vi "Patch data preview prototype.vi"(11 "Dataset path":path=path "C:/Users/Teo/Desktop/UCL Datasets/160915_13_48_57 FunctAcq-6 patches") -> ()   [LabVIEW 2017]
uses:
  Patch data preview/Typedefs/Patch viewer states.ctl
  Typedefs/Read Write Enum.ctl
panel:
  in  "Channel to load":enum16{"Red", "Green"}(ring)
  out "Slider at trial #":i32=11 format="Cycle: %.0f"
  in  "Scrollbar":i32(c297)=11
  out "Image":T1(plugin-control)
  in  "Number of rows to generate":i32=3
  # "C:\\Users\\Teo\\Desktop\\UCL Datasets\\160408_12_51_00-backwards jumps-Patches"
  # "This is the prototype patch data preview window. Its functionality will be integrated in the \"Window-Functional data editor.vi\"\nUpgrade to handle datasets with multiple trials."
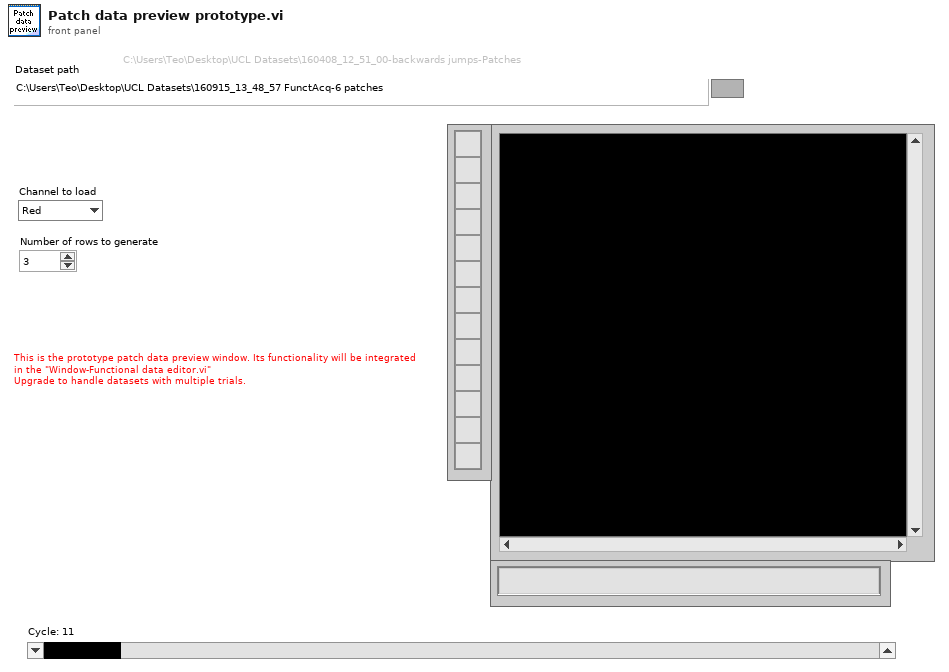
[diagram p1: front panel]
types:
  T1 = typedef "IMAQ Image.ctl" = refnum<image>
  T2 = typedef "Patch viewer states.ctl" = enum16{"Initialise", "Refresh", "Idle", "Error"}
  T3 = typedef "Read Write Enum.ctl" = enum16{"Read", "Write"}
  T4 = typedef "Patch viewer internal cluster.ctl" = cluster{"Image ref":T1, "Coordinates of montage positions":cluster{"X\n\nY":i32[]}[], "TDMS refs":refnum<k34>[], "Frames info":cluster{"Frame numbers used":i32[], "Frame position index":i32[]}, "Number of trials":i32, "Cycles in single trial":i32, "Total number of cycles":i32, "Number of patches":i32, "Pixels in a cycle":i32, "Patches info array":cluster{"Pixels in a patch":i32, "X size of patch":i32, "Y size of patch":i32}[], "error":errorcluster}
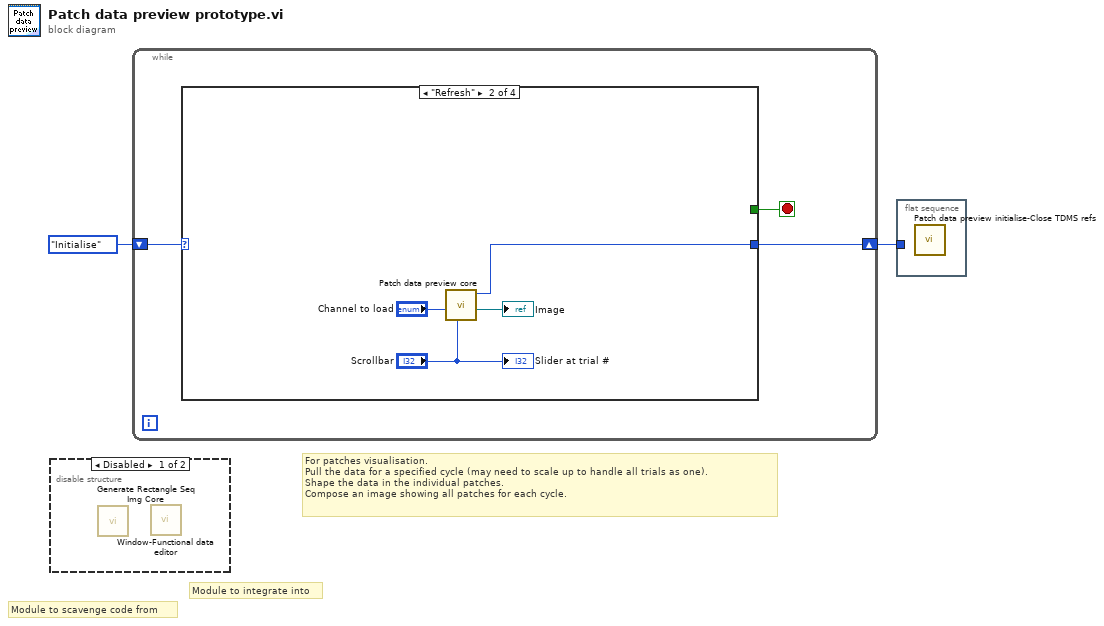
[diagram p0: block diagram]
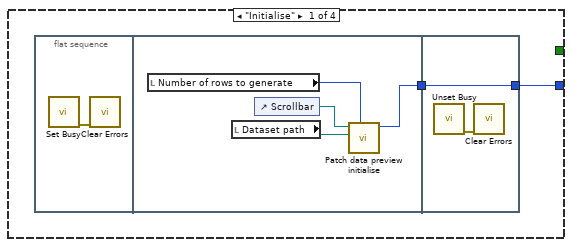
[diagram p3: hidden frame]
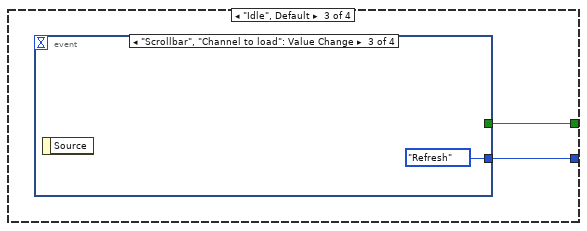
[diagram p4: hidden frame]
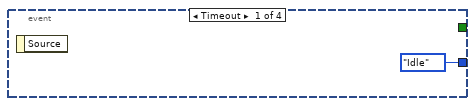
[diagram p5: hidden frame]
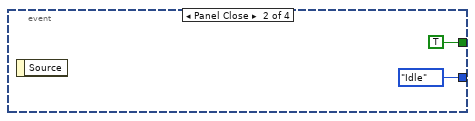
[diagram p6: hidden frame]
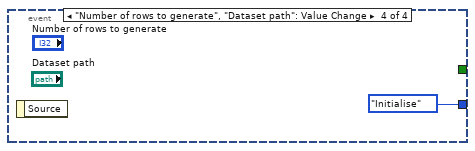
[diagram p7: hidden frame]
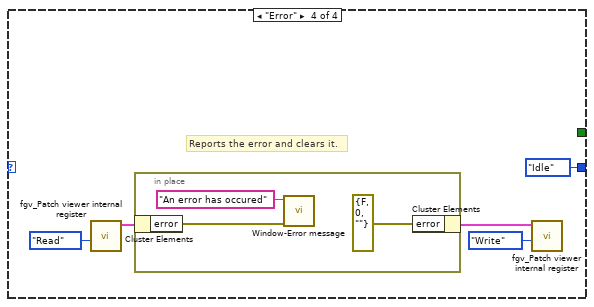
[diagram p8: hidden frame]
diagram:
  # "Module to integrate into"
  # "Module to scavenge code from"
  # "For patches visualisation.\nPull the data for a specified cycle (may need to scale up to handle all trials as one).\nShape the data in the individual patches.\nCompose an image showing all patches for each cycle."
  n1 = disable-structure shown="Disabled" {
    frame Disabled {
      n2 = call "Generate Rectangle Seq Img Core.vi"() -> ()  [unwired: 10 in, 2 out]
      n3 = call "Window-Functional data editor.vi"() -> ()  [unwired: 12 in]
    }
    frame Enabled {
    }
  }
  n4 = while {
    shift-right: [w3] -> w1
    shift-left: Patch_viewer_states."Initialise" ("States") -> [w5]
    stop <- w4 stop-if-true
    n5 = case shown="\"Refresh\"" w5 {
      tunnel: [_ _ w20 _] -> w4
      tunnel: [w7 w16 w19 Patch_viewer_states."Idle" ("States")] -> w3
      frame "Initialise" {
        n6 = flat-sequence {
          tunnel: [w10] -> w6
          tunnel: [w14] -> w7
          tunnel: w6 -> [w14]
          frame #0 {
            n7 = call <vilib>:"Set Busy.vi"() -> ("error out"=w8:errorcluster)  [unwired: 10 in, 1 out]
            n8 = call <vilib>:"Clear Errors.vi"("error in (no error)"=w8) -> ()  [unwired: 5 in, 2 out]
          }
          frame #1 {
            n9 = local read "Number of rows to generate"() -> (w9:i32)
            n10 = local read "Dataset path"() -> (w11:path)
            n11 = control-ref of="Scrollbar"() -> (w12:refnum<vi>)
            n12 = call "Patch data preview initialise.vi"("Number of rows to generate"=w9, "Dataset path"=w11, "Scrollbar ref"=w12) -> ("Next state"=w10:T2)  [unwired: 8 in]
          }
          frame #2 {
            n13 = call <vilib>:"Unset Busy.vi"() -> ("error out"=w13:errorcluster)  [unwired: 11 in]
            n14 = call <vilib>:"Clear Errors.vi"("error in (no error)"=w13) -> ()  [unwired: 5 in, 2 out]
          }
        }
      }
      frame "Refresh" {
        n15 = call "Patch data preview core.vi"("Global cycle number among all trials"="Scrollbar", "Channel to load"="Channel to load") -> ("Image ref (montage)"=→"Image":T1, "Next state"=w16:T2)  [unwired: 8 in]
        "Slider at trial #" <- "Scrollbar"
      }
      frame "Idle", Default {
        n16 = event shown="[2] \"Scrollbar\", \"Channel to load\": Value Change" {
          selector: _ -> [_ _ _ _]
          dyn-events: _ -> [_ _ _ _]
          timeout: _ -> [_ _ _ _]
          tunnel: [_ TRUE _ _] -> w20
          tunnel: [Patch_viewer_states."Idle" ("States") Patch_viewer_states."Idle" ("States") Patch_viewer_states."Refresh" ("States") Patch_viewer_states."Initialise" ("States")] -> w19
          event Timeout {
            n17 = event-data() -> ()  [unwired: 1 in, 1 out]
          }
          event Panel Close {
            n18 = event-data() -> ()  [unwired: 1 in, 1 out]
          }
          event "Scrollbar", "Channel to load": Value Change {
            n19 = event-data() -> ()  [unwired: 1 in, 1 out]
          }
          event "Number of rows to generate", "Dataset path": Value Change {
            n20 = event-data() -> ()  [unwired: 1 in, 1 out]
          }
        }
      }
      frame "Error" {
        # "Reports the error and clears it."
        n21 = call "fgv_Patch viewer internal register.vi"("Function"=Read_Write_Enum."Read") -> ("Registered setup"=w28:T4)  [unwired: 10 in]
        n22 = in-place {
          n23 = in-place-cluster #1(w28) -> ("error"=w33:errorcluster)
          n24 = call "Window-Error message.vi"("error in (no error)"=w33, "Message"="An error has occured") -> ()  [unwired: 9 in, 1 out]
          n25 = in-place-cluster #1("error"=errorcluster {"status"=FALSE, "code"=0, "source"=""} ("error out")) -> (w26:T4)
        }
        n26 = call "fgv_Patch viewer internal register.vi"("Function"=Read_Write_Enum."Write", "Registered setup"=w26) -> ()  [unwired: 9 in, 1 out]
      }
    }
  }
  n27 = flat-sequence {
    tunnel: w1 -> [_]
    frame #0 {
      n28 = call "Patch data preview initialise-Close TDMS refs.vi"() -> ()  [unwired: 11 in, 1 out]
    }
  }
